vi "Save_Benchmark_Results.vi"(6 "Header":string[](array[string]), 7 "file path (dialog if empty)":path, 11 "Execution Time":cluster{i32[], "FFT mean Exec Time":dbl[]}[](graph)=[{[100, 200, 300, 400, 500, 600, 700, 800, 900, 1000], "FFT mean Exec Time"=[0.20254379999823868, 0.18739450000066427, 0.1876723999994283, 0.1811310000011872, 0.18045799999890733, 0.19520859999829554, 0.2588984000030905, 0.3341770000006363, 0.42056009999942034, 0.5186259000001883]}, {[100, 200, 300, 400, 500, 600, 700, 800, 900, 1000], "FFT mean Exec Time"=[1.4655237999977544, 1.4558656999979576, 1.5842603999990388, 1.9962144999990414, 2.4267060999991372, 3.3026086000027135, 4.083992699997907, 9.061100799997803, 14.595555600000807, 18.715055600001506]}, {[100, 200, 300, 400, 500, 600, 700, 800, 900, 1000], "FFT mean Exec Time"=[0.12680180000097607, 0.49430969999957597, 1.1241387000009126, 2.0521574999984296, 3.3073327999991307, 4.815520899999683, 6.617998300000181, 8.800476899999921, 10.92705930000011, 13.463581899999554]}]) -> ()   [LabVIEW 2020]
uses:
  <vilib>/Utility/file.llb/Write Delimited Spreadsheet (string).vi
panel:
  out "new file path (Not A Path if cancelled)":path
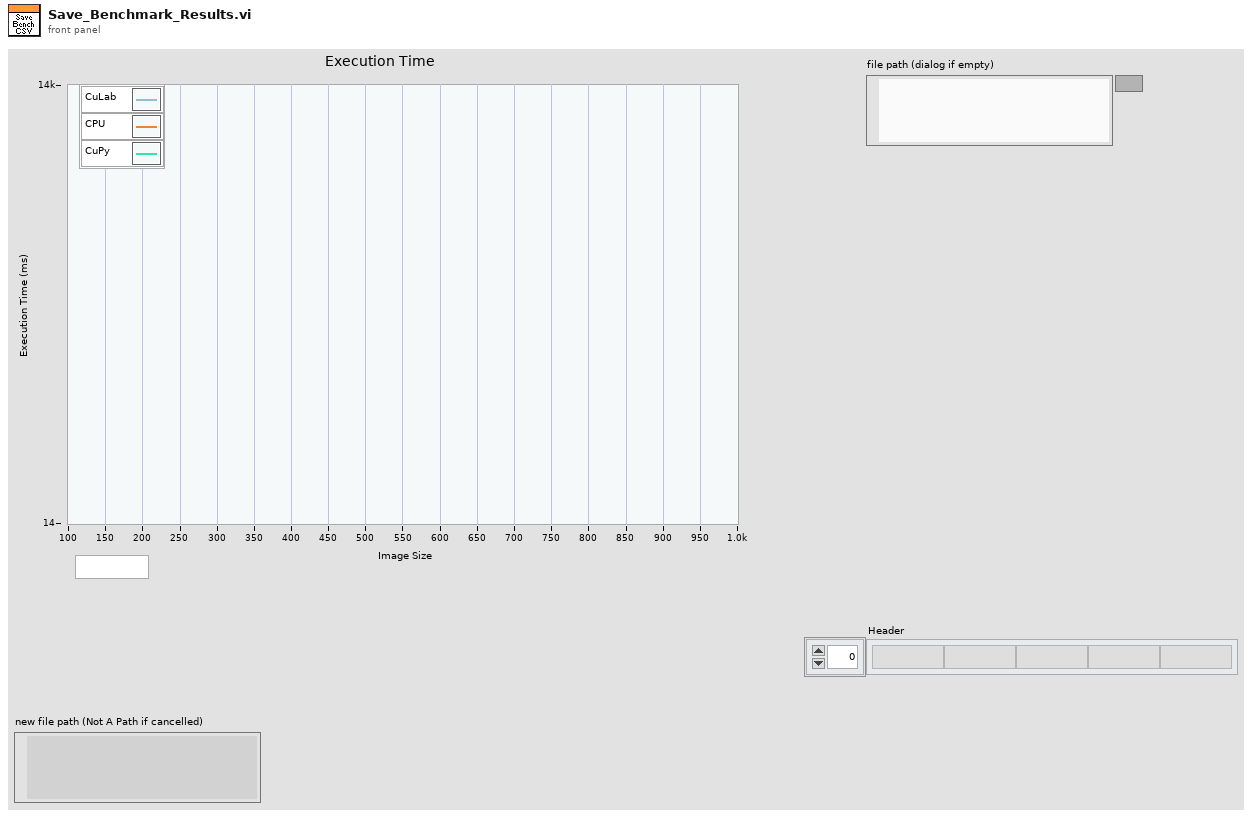
[diagram p1: front panel]
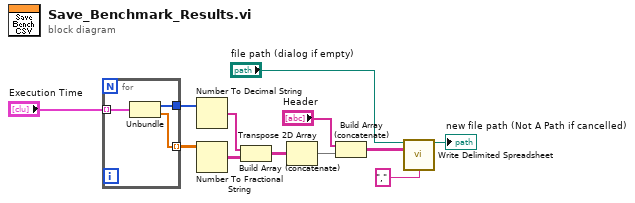
[diagram p0: block diagram]
diagram:
  n1 = for {
    tunnel: "Execution Time" -> [w15] mode=indexing
    tunnel: [w14] -> w11 mode=indexing
    tunnel: [w13] -> w12
    n2 = Unbundle(w15) -> (w13:i32[], "FFT mean Exec Time"=w14:dbl[])
  }
  n3 = Number To Decimal String(number=w12) -> (decimal integer string=w10:string[])  [unwired: 1 in]
  n4 = Number To Fractional String(number=w11) -> (F-format string=w9:string[][])  [unwired: 3 in]
  n5 = Build Array (concatenate)(w10, w9) -> (w8:string[][])
  n6 = Transpose 2D Array(2D array=w8) -> (transposed array=w7:string[][])
  n7 = Build Array (concatenate)("Header", w7) -> (w4:string[][])
  n8 = call-poly <vilib>:"Write Delimited Spreadsheet.vi"("file path (dialog if empty)"="file path (dialog if empty)", "2D data"=w4, "delimiter (\\t)"="," ("delimiter (\\t)")) -> ("new file path (Not A Path if cancelled)"=→"new file path (Not A Path if cancelled)":path)  [unwired: 11 in, 1 out]
